vi "readRelaySpec.vi"(1 "RelaySpec":T1) -> (0 "Relay Status":bool)   [LabVIEW 2011]
uses:
  relaySpec.ctl
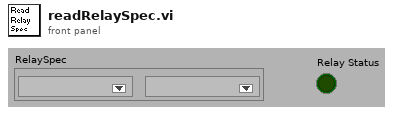
[diagram p1: front panel]
types:
  T1 = typedef "relaySpec.ctl" = cluster{"Card Index":u16, "Relay Index":u16}
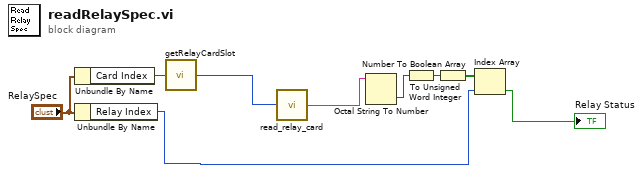
[diagram p0: block diagram]
diagram:
  n1 = Unbundle By Name("RelaySpec") -> ("Card Index"=w4:u16)
  n2 = Unbundle By Name("RelaySpec") -> ("Relay Index"=w2:u16)
  n3 = call "getRelayCardSlot.vi"("Relay Card Index"=w4) -> ("Slot"=w1:u16)
  n4 = call "read_relay_card.vi"("Slot"=w1) -> ("data"=w6:string)
  n5 = Octal String To Number(4:w6) -> (0:w7:u32)  [unwired: 3 out]
  n6 = To Unsigned Word Integer(number=w7) -> (unsigned 16bit integer=w8:u16)
  n7 = Number To Boolean Array(number=w8) -> (Boolean array=w9:bool[])
  n8 = Index Array(array=w9, index=w2) -> (element=→"Relay Status":bool)
